vi "Copy Value.vi"(10 "From":refnum<class "Type.lvclass">, 11 "Boolean in":refnum<class "Boolean.lvclass">) -> (2 "error out":errorcluster, 3 "Boolean out":refnum<class "Boolean.lvclass">)   [LabVIEW 2020, in "Conditu2.lvlib" / "Columns.lvlib" / "Boolean.lvclass"]
uses:
  Boolean.lvclass
  C:/dev/lv20CE/lv-conditum-tools/Conditum-Clone/Columns/Type/Type.lvclass
  Type/Type.lvclass
  Boolean.lvclass/Boolean.ctl
  Type/Type.lvclass/Type.ctl
  Type/Clear NULL.vi
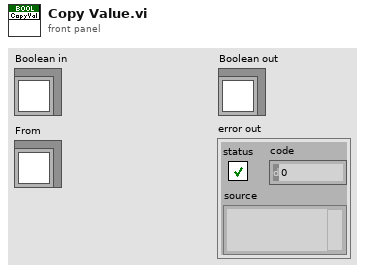
[diagram p1: front panel]
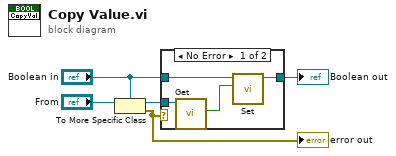
[diagram p0: block diagram]
diagram:
  n1 = To More Specific Class(target class="Boolean in", reference="From") -> (specific class reference=w4:refnum<class "Boolean.lvclass">, error out=w1:errorcluster)  [unwired: 1 in]
  "error out" <- w1
  n2 = case shown="No Error" w1 {
    tunnel: w4 -> [w9 _]
    tunnel: "Boolean in" -> [w7 w10]
    tunnel: [w6 w10] -> w2
    frame No Error {
      n3 = call "Get.vi"("Boolean in"=w9) -> ("Value"=w8:bool)  [unwired: 10 in]
      n4 = call "Set.vi"("Value"=w8, "Boolean in"=w7) -> ("Boolean out"=w6:refnum<class "Boolean.lvclass">)  [unwired: 9 in]
    }
    frame Error {
    }
  }
  "Boolean out" <- w2
